vi "stop.vi"(4 "error in (no error)":errorcluster, 6 "Request data":variant, 7 "Python session in":refnum<k35>) -> (0 "error out":errorcluster, 2 "Response data":variant, 3 "Python session out":refnum<k35>)   [LabVIEW 2018]
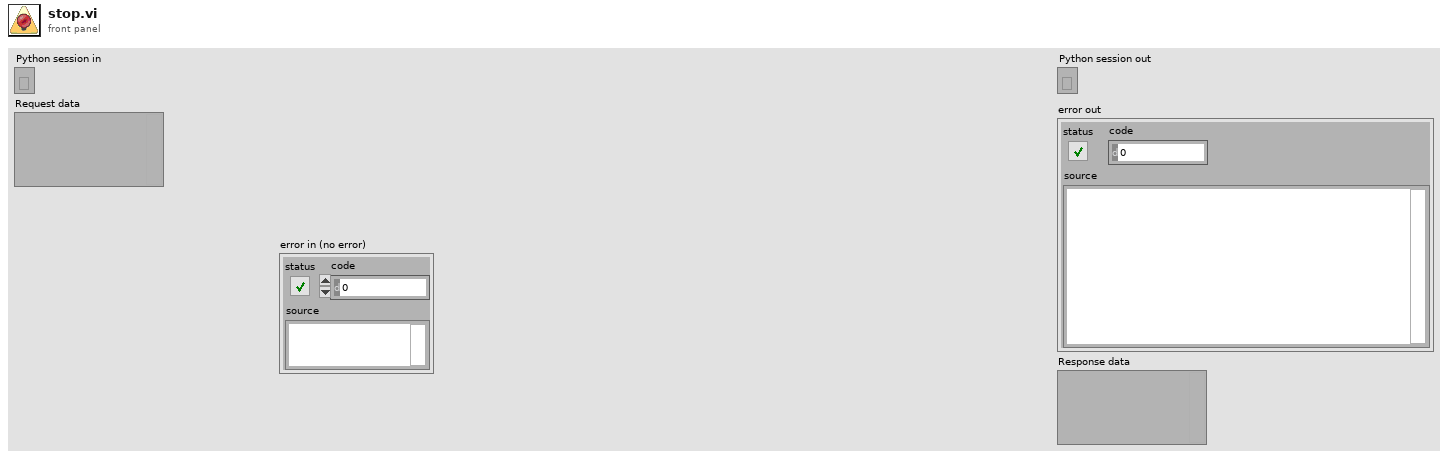
[diagram p1: front panel]
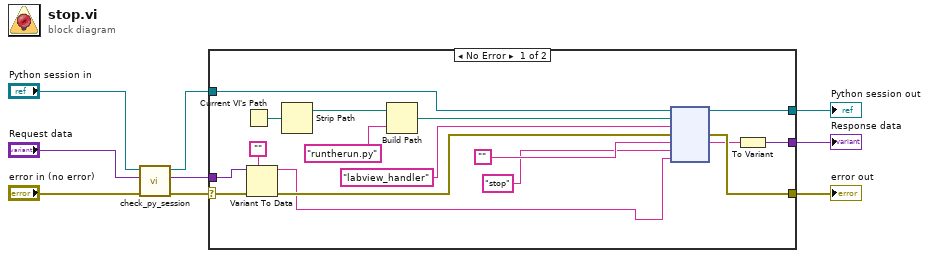
[diagram p0: block diagram]
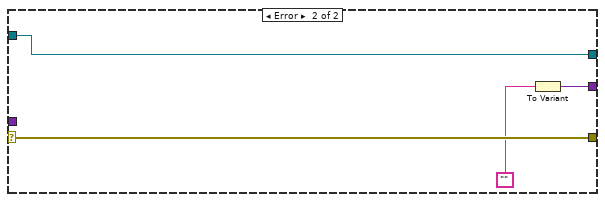
[diagram p2: hidden frame]
diagram:
  n1 = call "check_py_session.vi"("error in"="error in (no error)", "Request data"="Request data", "Python session in"="Python session in") -> ("error out"=w3:errorcluster, "Response data"=w4:variant, "Python session out"=w5:refnum<k35>)  [unwired: 2 in]
  n2 = case shown="No Error" w3 {
    selector: w3 -> [w16 w30]
    tunnel: w5 -> [w26 w29]
    tunnel: [w19 w29] -> w9
    tunnel: w4 -> [w17 _]
    tunnel: [w14 w30] -> w2
    tunnel: [w12 w27] -> w1
    frame No Error {
      n3 = Current VI's Path() -> (path=w21:path)
      n4 = Variant To Data(error in=w16, type="", Variant=w17) -> (data=w11:string, error out=w15:errorcluster)
      n5 = Strip Path(path=w21) -> (stripped path=w20:path)  [unwired: 1 out]
      n6 = Build Path(base path=w20, name or relative path="runtherun.py") -> (appended path=w23:path)
      n7 = node(w26, w23, "labview_handler" ("function name"), w15, "", "stop", w11) -> (w19:refnum<k35>, w14:errorcluster, w13:string)  [unwired: 2 in, 2 out]
      n8 = To Variant(anything=w13) -> (Variant=w12:variant)
    }
    frame Error {
      n9 = To Variant(anything="") -> (Variant=w27:variant)
    }
  }
  "error out" <- w2
  "Python session out" <- w9
  "Response data" <- w1
